vi "Configure.vi"(8 "error in (no error)":errorcluster, 10 "Msg in":T1, 11 "FakePressureController in":refnum<class "SMC100.lvclass">) -> (0 "error out":errorcluster, 1 "new command":string, 2 "Msg out":T1, 3 "FakePressureController out":refnum<class "SMC100.lvclass">)   [LabVIEW 2020, in "SMC100.lvclass"]
uses:
  SMC100.lvclass
  DriverMsg.ctl
  SMC100.lvclass/SMC100.ctl
  OnOffTypeDef.ctl
  CompressAndUpdate(Numeric).vi
  CompressAndUpdate(Enum).vi
  source/Device Drivers/BaseDriver/BaseDriver.lvclass
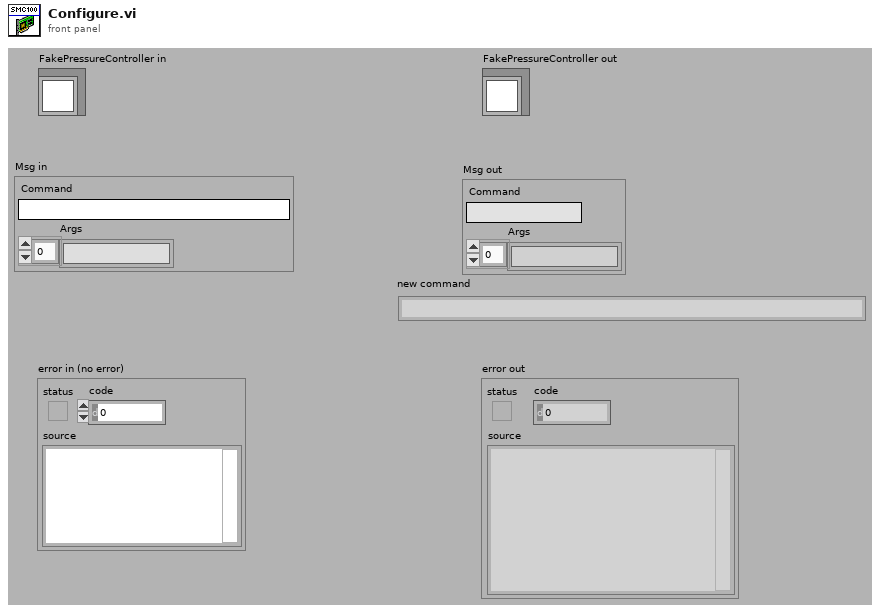
[diagram p1: front panel]
types:
  T1 = typedef "DriverMsg.ctl" = cluster{"Command":string, "Args":string[]}
  T2 = cluster{"VisaResourceName":string, "DeviceName":string, i32, "error out":errorcluster}
  T3 = cluster{"VISA resource name":refnum<visa-resource-name>, "Device name":string, "Controller address":i32, "error":errorcluster}
  T4 = typedef "OnOffTypeDef.ctl" = enum16{"off", "on"}
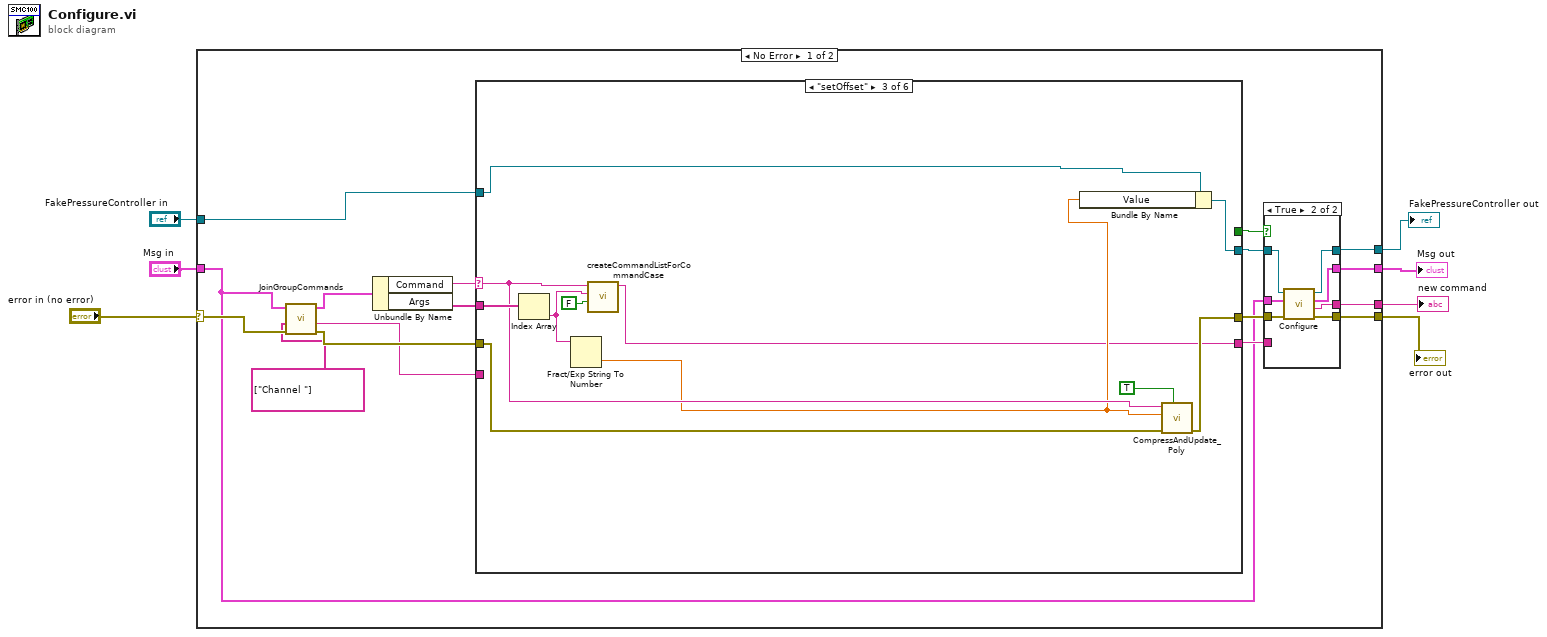
[diagram p0: block diagram]
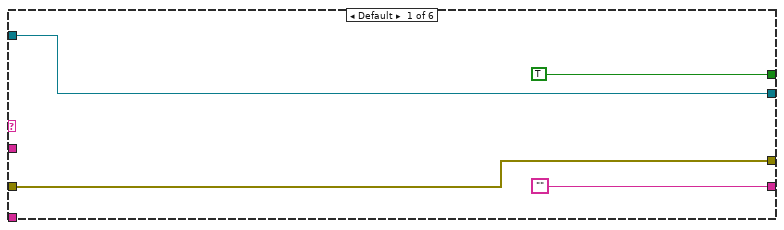
[diagram p3: hidden frame]
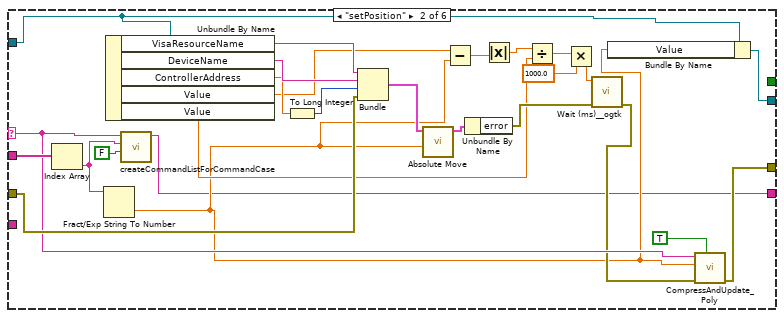
[diagram p4: hidden frame]
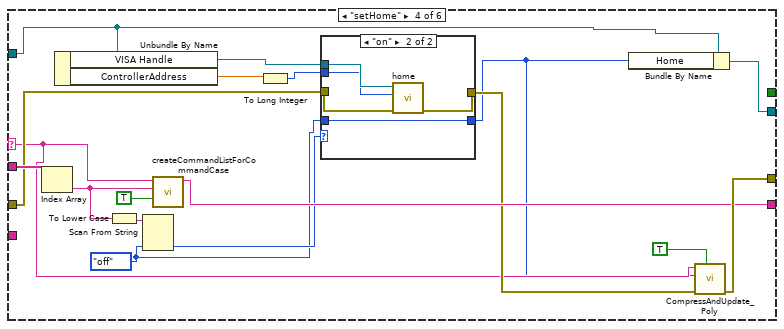
[diagram p5: hidden frame]
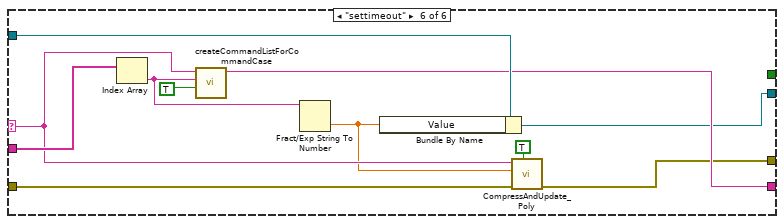
[diagram p8: hidden frame]
diagram:
  n1 = case shown="No Error" "error in (no error)" {
    selector: "error in (no error)" -> [w13 w117]
    tunnel: "FakePressureController in" -> [w15 w115]
    tunnel: [w23 w115] -> w4
    tunnel: [w21 w117] -> w1
    tunnel: "Msg in" -> [w10 w116]
    tunnel: [w19 w116] -> w3
    tunnel: [w17 _] -> w2
    frame No Error {
      n2 = call "JoinGroupCommands.vi"("error in (no error)"=w13, "Seperator between var name and chan num"=string[] ["Channel "], "Msg in"=w10) -> ("error out"=w12:errorcluster, "Seperator out"=w9:string, "Msg out"=w11:T1)  [unwired: 5 in, 1 out]
      n3 = Unbundle By Name(w11) -> ("Command"=w16:string, "Args"=w14:string[])
      n4 = case shown="\"setOffset\"" w16 {
        selector: w16 -> [_ w54 w72 w78 _ w110]
        tunnel: w12 -> [w38 w58 w66 w84 w102 w108]
        tunnel: w14 -> [_ w64 w75 w94 _ w112]
        tunnel: w15 -> [w39 w42 w69 w86 w103 w114]
        tunnel: [w39 w41 w68 w91 w103 w106] -> w24
        tunnel: ["" ("Complete") w40 w67 w87 _ w111] -> w18
        tunnel: [w38 w53 w71 w92 w102 w107] -> w22
        tunnel: [TRUE _ _ _ _ _] -> w20
        tunnel: w9 -> [_ _ _ _ _ _]
        frame Default {
        }
        frame "setPosition" {
          n5 = Index Array(array=w64) -> (element=w63:string)  [unwired: 1 in]
          n6 = Fract/Exp String To Number(string=w63) -> (number=w43:dbl)  [unwired: 3 in, 1 out]
          n7 = Unbundle By Name(w42) -> ("VisaResourceName"=w62:string, "DeviceName"=w61:string, "ControllerAddress"=w60:dbl, "Value"=w50:dbl, "Value"=w47:dbl)
          n8 = call "createCommandListForCommandCase.vi"("immediate Check (only once)"=FALSE, "setvalue"=w63, "command"=w54) -> ("new commands"=w40:string)  [unwired: 8 in]
          n9 = To Long Integer(number=w60) -> (32bit integer=w59:i32)
          n10 = Bundle("VisaResourceName"=w62, "DeviceName"=w61, w59, "error out"=w58) -> (w57:T2)  [unwired: 1 in]
          n11 = call "Absolute Move.vi"("Target position"=w43, "Connection Cluster in"=w57) -> ("Connection Cluster out"=w56:T3)  [unwired: 5 in, 2 out]
          n12 = Subtract(x=w50, y=w43) -> (x-y=w49:dbl)
          n13 = Unbundle By Name(w56) -> ("error"=w52:errorcluster)
          n14 = Absolute Value(x=w49) -> (abs(x)=w48:dbl)
          n15 = Divide(x=w48, y=w47) -> (x/y=w46:dbl)
          n16 = Multiply(x=w46, y=1000.0) -> (x*y=w44:dbl)
          n17 = call "Wait (ms)__ogtk.vi"("error in (no error)"=w52, "milliseconds to wait"=w44) -> ("error out"=w51:errorcluster)  [unwired: 8 in, 1 out]
          n18 = Bundle By Name(cluster=w42, "Value"=w43) -> (w41:refnum<class "SMC100.lvclass">)
          n19 = call-poly "CompressAndUpdate_Poly.vi"("force CVT update (false)"=TRUE, "error in"=w51, "Numeric"=w43, "command or variable name"=w54) -> ("error out"=w53:errorcluster)  [unwired: 7 in]
        }
        frame "setOffset" {
          n20 = Index Array(array=w75) -> (element=w74:string)  [unwired: 1 in]
          n21 = Fract/Exp String To Number(string=w74) -> (number=w70:dbl)  [unwired: 3 in, 1 out]
          n22 = call "createCommandListForCommandCase.vi"("immediate Check (only once)"=FALSE, "setvalue"=w74, "command"=w72) -> ("new commands"=w67:string)  [unwired: 8 in]
          n23 = Bundle By Name(cluster=w69, "Value"=w70) -> (w68:refnum<class "SMC100.lvclass">)
          n24 = call-poly "CompressAndUpdate_Poly.vi"("force CVT update (false)"=TRUE, "error in"=w66, "Numeric"=w70, "command or variable name"=w72) -> ("error out"=w71:errorcluster)  [unwired: 7 in]
        }
        frame "setHome" {
          w79 = OnOffTypeDef."off" ("Settings.Trigger")
          n25 = Index Array(array=w94) -> (element=w88:string)  [unwired: 1 in]
          n26 = Unbundle By Name(w86) -> ("VISA Handle"=w85:refnum<visa-resource-name>, "ControllerAddress"=w82:dbl)
          n27 = To Lower Case(string=w88) -> (all lower case string=w89:string)
          n28 = Scan From String(input string=w89, default 1=w79) -> (output 1=w80:T4)  [unwired: 3 in, 3 out]
          n29 = call "createCommandListForCommandCase.vi"("immediate Check (only once)"=TRUE, "setvalue"=w88, "command"=w78) -> ("new commands"=w87:string)  [unwired: 8 in]
          n30 = To Long Integer(number=w82) -> (32bit integer=w81:i32)
          n31 = case shown="\"on\"" w80 {
            tunnel: w85 -> [_ w101]
            tunnel: w84 -> [w96 w100]
            tunnel: [w96 w99] -> w83
            tunnel: w81 -> [_ w98]
            tunnel: w79 -> [w95 w97]
            tunnel: [w95 w97] -> w77
            frame "off", Default {
            }
            frame "on" {
              n32 = call "home.vi"("error in"=w100, "Axis in"=w98, "VISA Handle in"=w101) -> ("error out"=w99:errorcluster)  [unwired: 3 in, 3 out]
            }
          }
          n33 = Bundle By Name(cluster=w86, "Home"=w77) -> (w91:refnum<class "SMC100.lvclass">)
          n34 = call-poly "CompressAndUpdate_Poly.vi"("force CVT update (false)"=TRUE, "error in"=w83, "enum variant"=w77, "command or variable name"=w78) -> ("error out"=w92:errorcluster)  [unwired: 7 in]
        }
        frame "Abort" {
        }
        frame "settimeout" {
          n35 = Index Array(array=w112) -> (element=w105:string)  [unwired: 1 in]
          n36 = call "createCommandListForCommandCase.vi"("immediate Check (only once)"=TRUE, "setvalue"=w105, "command"=w110) -> ("new commands"=w111:string)  [unwired: 8 in]
          n37 = Fract/Exp String To Number(string=w105) -> (number=w104:dbl)  [unwired: 3 in, 1 out]
          n38 = Bundle By Name(cluster=w114, "Value"=w104) -> (w106:refnum<class "SMC100.lvclass">)
          n39 = call-poly "CompressAndUpdate_Poly.vi"("force CVT update (false)"=TRUE, "error in"=w108, "Numeric"=w104, "command or variable name"=w110) -> ("error out"=w107:errorcluster)  [unwired: 7 in]
        }
      }
      n40 = case shown="True" w20 {
        tunnel: w24 -> [w26 w35]
        tunnel: [w26 w34] -> w23
        tunnel: [w27 w33] -> w17
        tunnel: w22 -> [w25 w32]
        tunnel: [w25 w31] -> w21
        tunnel: w10 -> [w28 w30]
        tunnel: [w28 w29] -> w19
        tunnel: w18 -> [w27 _]
        frame False {
        }
        frame True {
          n41 = call-parent "Configure.vi"("error in (no error)"=w32, "Msg in"=w30, "BaseDriver in"=w35) -> ("error out"=w31:errorcluster, "new command"=w33:string, "Msg out"=w29:T1, "BaseDriver out"=w34:refnum<class "SMC100.lvclass">)  [unwired: 5 in]
        }
      }
    }
    frame Error {
    }
  }
  "error out" <- w1
  "FakePressureController out" <- w4
  "new command" <- w2
  "Msg out" <- w3
